vi "Transcript Example Arduino Blink LED.vi"() -> ()   [LabVIEW 2018]
panel:
  out "transcripted code":string
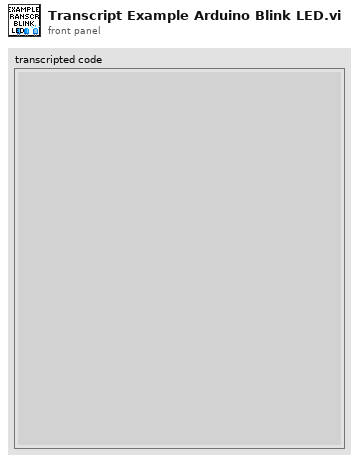
[diagram p1: front panel]
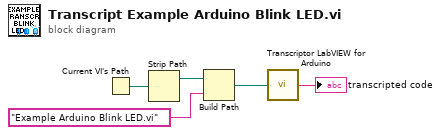
[diagram p0: block diagram]
diagram:
  n1 = Current VI's Path() -> (path=w5:path)
  n2 = Strip Path(path=w5) -> (stripped path=w4:path)  [unwired: 1 out]
  n3 = Build Path(base path=w4, name or relative path="Example Arduino Blink LED.vi") -> (appended path=w2:path)
  n4 = call "Transcriptor LabVIEW for Arduino.vi"("vi path"=w2) -> ("transcripted code"=→"transcripted code":string)
